vi "Update Value by Name.vi"(7 "Overwrite? (F)":bool, 8 "error in (no error)":errorcluster, 9 "Value":variant, 10 "Name":string, 11 "Values in":refnum<class "Values.lvclass">) -> (0 "error out":errorcluster, 3 "Values out":refnum<class "Values.lvclass">)   [LabVIEW 2020, in "HTTP Server.lvlib" / "Values.lvclass"]
uses:
  Values.lvclass
  Values.lvclass/Values.ctl
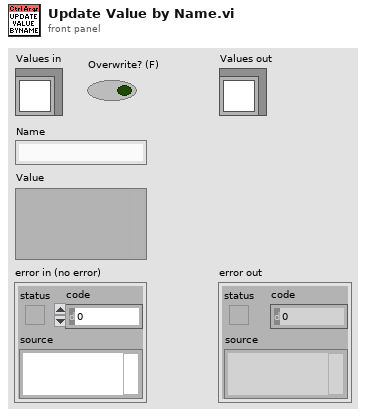
[diagram p1: front panel]
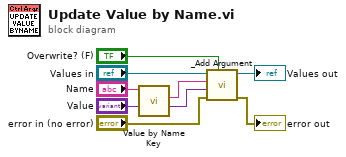
[diagram p0: block diagram]
diagram:
  n1 = call "Value by Name Key.vi"("Value Name In"="Name") -> ("Value by Name Key"=w3:string)  [unwired: 9 in, 1 out]
  n2 = call "_Add Argument.vi"("Overwrite? (F)"="Overwrite? (F)", "error in (no error)"="error in (no error)", "Value"="Value", "Name"=w3, "Arguments in"="Values in") -> ("error out"=→"error out":errorcluster, "Arguments out"=→"Values out":refnum<class "Values.lvclass">)  [unwired: 5 in]
